vi "Write Experiment Folder.vi"(8 "error in (no error)":errorcluster, 10 "Experiment Folder":string, 11 "Control Experiment":refnum<class "Control Experiment.lvclass">) -> (0 "error out":errorcluster, 3 "Control Experiment out":refnum<class "Control Experiment.lvclass">)   [LabVIEW 2016, in "Control Experiment.lvclass"]
uses:
  Control Experiment.lvclass
  Control Experiment.lvclass/Control Experiment.ctl
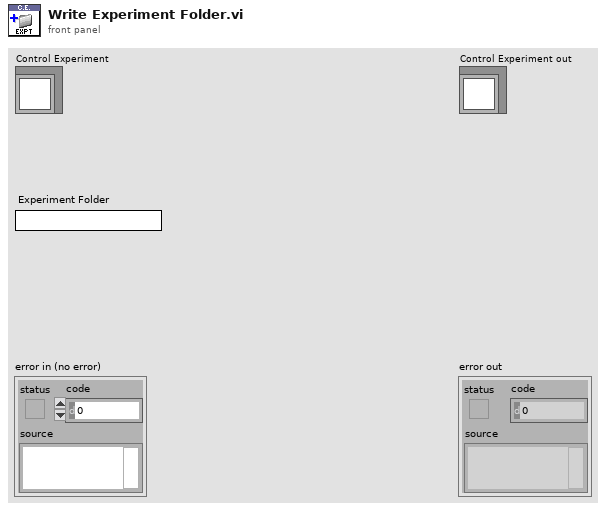
[diagram p1: front panel]
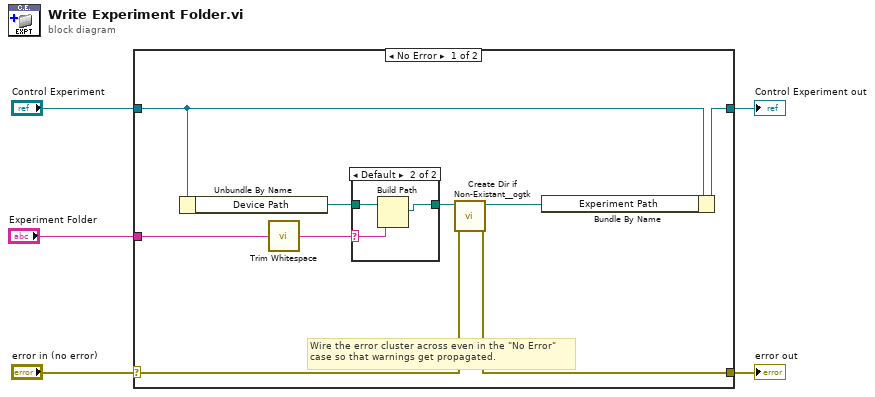
[diagram p0: block diagram]
diagram:
  n1 = case shown="No Error" "error in (no error)" {
    selector: "error in (no error)" -> [w7 w20]
    tunnel: [w6 w20] -> w4
    tunnel: [w13 w19] -> w2
    tunnel: "Control Experiment" -> [w14 w19]
    tunnel: "Experiment Folder" -> [w11 _]
    frame No Error {
      # "Wire the error cluster across even in the \"No Error\"\ncase so that warnings get propagated."
      n2 = Unbundle By Name(w14) -> ("Device Path"=w12:path)
      n3 = call <vilib>:"Trim Whitespace.vi"("string"=w11) -> ("trimmed string"=w10:string)  [unwired: 1 in]
      n4 = case shown="Default" w10 {
        selector: w10 -> [_ w17]
        tunnel: [w15 w16] -> w9
        tunnel: w12 -> [w15 w18]
        frame "" {
        }
        frame Default {
          n5 = Build Path(base path=w18, name or relative path=w17) -> (appended path=w16:path)
        }
      }
      n6 = call <userlib>:"Create Dir if Non-Existant__ogtk.vi"("error in (no error)"=w7, "Directory Path"=w9) -> ("error out"=w6:errorcluster, "dup Directory Path"=w8:path)  [unwired: 7 in, 1 out]
      n7 = Bundle By Name(cluster=w14, "Experiment Path"=w8) -> (w13:refnum<class "Control Experiment.lvclass">)
    }
    frame Error {
    }
  }
  "error out" <- w4
  "Control Experiment out" <- w2
